vi "Restore Permissions.vi"(7 "Delay":u32=10 format="%.0fms", 8 "Error In":errorcluster, 10 "View only":bool, 11 "File Path":path) -> (0 "Error Out":errorcluster, 1 "standard error":string, 2 "standard output":string, 3 "Duplicate File Path":path)   [LabVIEW 2019]
panel:
  out "New group":string
  out "New owner":string
  out "New permissions":i16
  out "Old group":string
  out "Old owner":string
  out "Old permissions":i16
  out "return code":i32
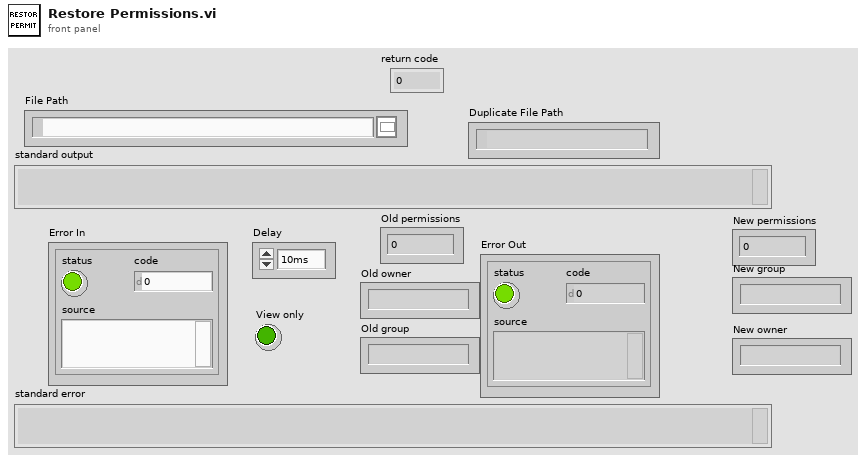
[diagram p1: front panel]
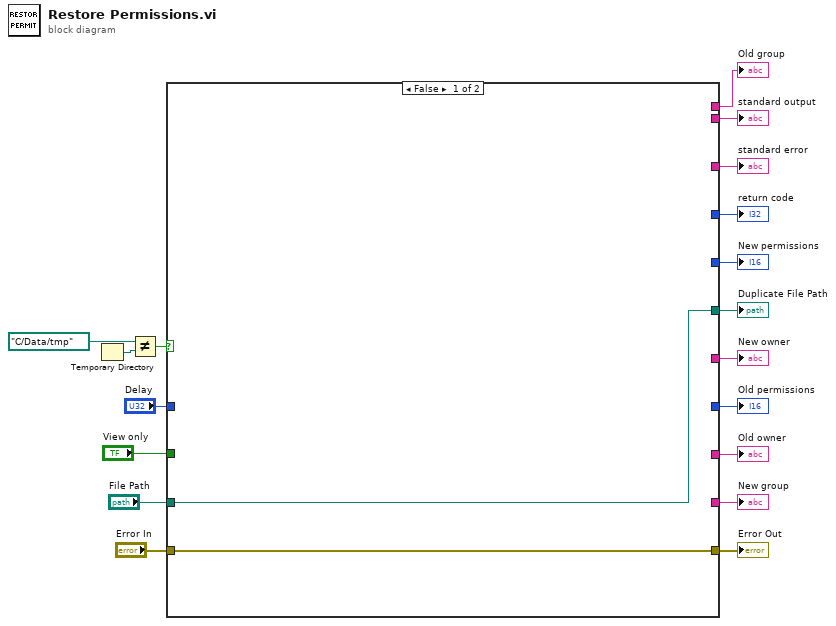
[diagram p0: block diagram]
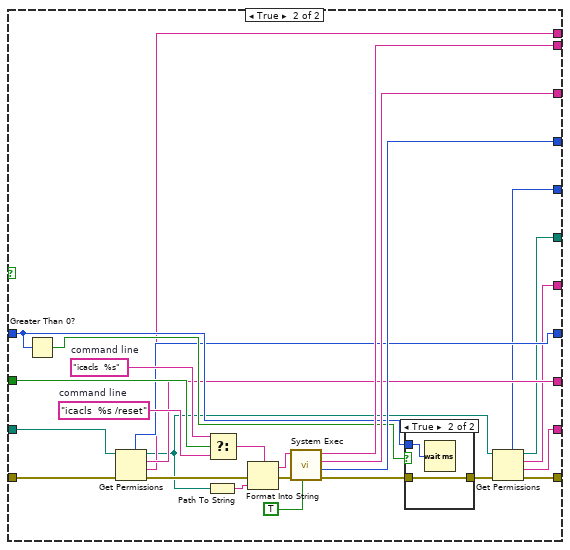
[diagram p2: hidden frame]
diagram:
  n1 = Temporary Directory() -> (w1:path)
  n2 = Not Equal?(x=path "C:/Data/tmp", y=w1) -> (x != y?=w2:bool)
  n3 = case shown="False" w2 {
    tunnel: [_ w44] -> w18
    tunnel: [_ w43] -> w17
    tunnel: [_ w42] -> w16
    tunnel: "Delay" -> [_ w39]
    tunnel: "View only" -> [_ w38]
    tunnel: "Error In" -> [w19 w34]
    tunnel: [_ w31] -> w12
    tunnel: "File Path" -> [w20 w30]
    tunnel: [_ w29] -> w10
    tunnel: [_ w28] -> w9
    tunnel: [w19 w26] -> w8
    tunnel: [w20 w24] -> w7
    tunnel: [_ w23] -> w6
    tunnel: [_ w22] -> w5
    tunnel: [_ w21] -> w4
    frame False {
    }
    frame True {
      w36 = "icacls  %s"  # command line
      w37 = "icacls  %s /reset"  # command line
      n4 = Greater Than 0?(x=w39) -> (x > 0?=w40:bool)
      n5 = Get Permissions(8:w34, 11:w30) -> (0:w33:errorcluster, 1:w28:string, 2:w29:string, 3:w25:path, 5:w31:i16)
      n6 = Path To String(path=w25) -> (string=w47:string)
      n7 = Select(t=w36, s=w38, f=w37) -> (s? t:f=w35:string)
      n8 = Format Into String(format string=w35, error in=w33, w47) -> (resulting string=w46:string, error out=w32:errorcluster)  [unwired: 1 in]
      n9 = call <vilib>:"System Exec.vi"("run minimized? (F)"=TRUE, "error in (no error)"=w32, "command line"=w46) -> ("error out"=w41:errorcluster, "return code"=w42:i32, "standard error"=w43:string, "standard output"=w44:string)  [unwired: 3 in, 2 out]
      n10 = case shown="True" w40 {
        tunnel: w41 -> [w48 w50]
        tunnel: [w48 w50] -> w27
        tunnel: w39 -> [_ w49]
        frame False {
        }
        frame True {
          n11 = Wait (ms)(milliseconds to wait=w49) -> ()  [unwired: 1 out]
        }
      }
      n12 = Get Permissions(8:w27, 11:w25) -> (0:w26:errorcluster, 1:w21:string, 2:w22:string, 3:w24:path, 5:w23:i16)
    }
  }
  "Error Out" <- w8
  "Duplicate File Path" <- w7
  "standard output" <- w18
  "standard error" <- w17
  "return code" <- w16
  "Old permissions" <- w12
  "Old owner" <- w10
  "Old group" <- w9
  "New permissions" <- w6
  "New owner" <- w5
  "New group" <- w4
